vi "FGV_Error Handler_Log Error.vi"(8 "error in (no error)":errorcluster, 9 "Classification":T1, 10 "Current Account":i32, 11 "Refnum in":refnum<k1>) -> (3 "Refnum out":refnum<k1>)   [LabVIEW 2012]
uses:
  DataType/FGV_Error Handler_Classification.ctl
  DataType/FGV_Error Handler_Error log.ctl
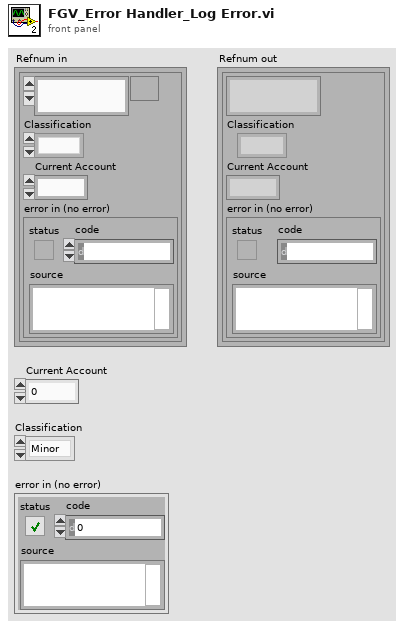
[diagram p1: front panel]
types:
  T1 = typedef "FGV_Error Handler_Classification.ctl" = enum16{"Minor", "Session", "System"}
  T2 = typedef "FGV_Error Handler_Error log.ctl" = cluster{timestamp, "Classification":T1, "Current Account":i32, "error in (no error)":errorcluster}
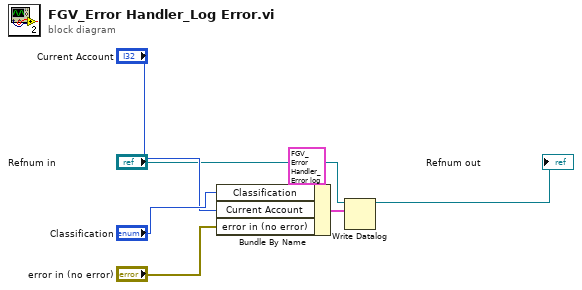
[diagram p0: block diagram]
diagram:
  n1 = Bundle By Name(cluster=T2 {timestamp(0 s since 1904-01-01), "Classification"=enum."Minor", "Current Account"=0, "error in (no error)"={"status"=FALSE, "code"=0, "source"=""}} ("record(s)"), "Classification"="Classification", "Current Account"="Current Account", "error in (no error)"="error in (no error)") -> (w4:T2)
  n2 = Write Datalog(6:w4, 7:"Refnum in") -> (3:→"Refnum out":refnum<k1>)  [unwired: 1 in, 1 out]
